vi "Add Project Item.vi"(8 "error in (no error)":errorcluster, 10 "Folder Location Ref":refnum<vi>, 11 "Module Loop in":refnum<class "Module Loop.lvclass">) -> (0 "error out":errorcluster, 3 "Module Loop out":refnum<class "Module Loop.lvclass">)   [LabVIEW 2025, in "Module Loop.lvclass"]
uses:
  Module Loop.lvclass
  Module Loop.lvclass/Module Loop.ctl
  Module/Module/Module.lvclass
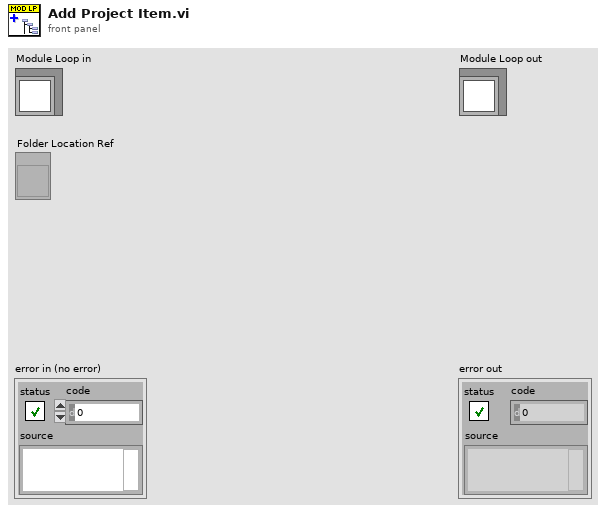
[diagram p1: front panel]
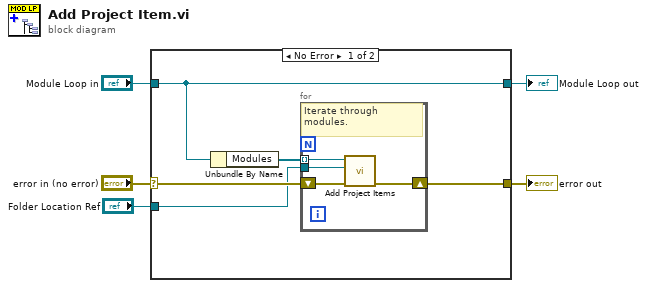
[diagram p0: block diagram]
diagram:
  n1 = case shown="No Error" "error in (no error)" {
    selector: "error in (no error)" -> [w9 w15]
    tunnel: [w8 w15] -> w4
    tunnel: "Module Loop in" -> [w7 w16]
    tunnel: [w7 w16] -> w2
    tunnel: "Folder Location Ref" -> [w6 _]
    frame No Error {
      n2 = Unbundle By Name(w7) -> ("Modules"=w10:refnum<class "Module.lvclass">[])
      n3 = for {
        tunnel: w10 -> [w14] mode=indexing
        shift-right: [w12] -> w8
        shift-left: w9 -> [w13]
        tunnel: w6 -> [w11]
        # "Iterate through modules."
        n4 = call-dynamic "Add Project Items.vi"("error in (no error)"=w13, "Folder Location Ref"=w11, "Module in"=w14) -> ("error out"=w12:errorcluster)  [unwired: 7 in, 1 out]
      }
    }
    frame Error {
    }
  }
  "error out" <- w4
  "Module Loop out" <- w2
